vi "ListThisLevelDependencies.vi"(8 "error in (no error)":errorcluster, 11 "SMO in":refnum<class "SMO.lvclass">) -> (0 "error out":errorcluster, 2 "[My Dependencies]":refnum<class "SMO.lvclass">[](array[class]), 3 "SMO out":refnum<class "SMO.lvclass">)   [LabVIEW 2021, in "smo.lvlib" / "SMO.lvclass"]
uses:
  SMO.lvclass
  SMO.lvclass/SMO.ctl
  Private/GetDependencies.vi
  Support/Attribute.Dependencies/List Dependencies.vi
  Private/GetVariant(Attr).vi
  Private/ReftoDVR--SMO.vi
  Support/Attribute.Dependencies/Get GUIDs.vi
  isStateMachineObject.vi
  Support/Attribute.Dependencies/Attribute.Dependencies.lvclass
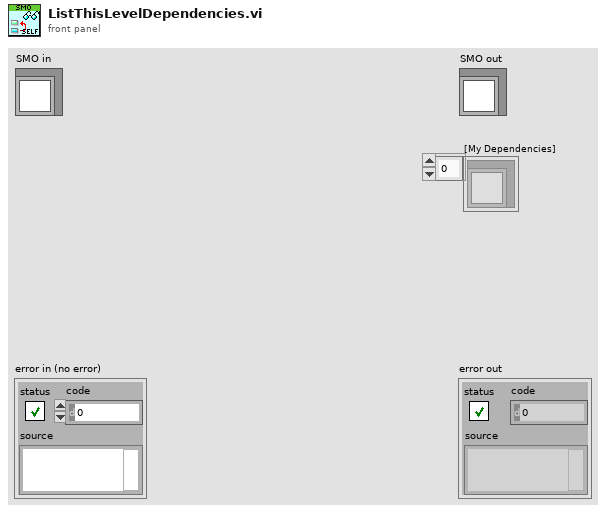
[diagram p1: front panel]
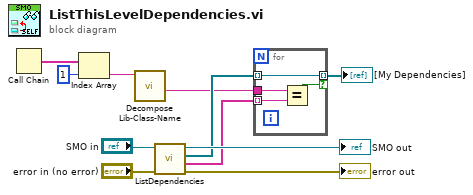
[diagram p0: block diagram]
diagram:
  n1 = Call Chain() -> (call chain=w11:string[])
  n2 = Index Array(array=w11, index=1) -> (element=w2:string)
  n3 = call "Decompose Lib-Class-Name.vi"("Qualified Name"=w2) -> ("className"=w1:string)  [unwired: 6 in, 4 out]
  n4 = call "ListDependencies.vi"("error in (no error)"="error in (no error)", "SMO in"="SMO in") -> ("error out"=→"error out":errorcluster, "Level"=w4:string[], "[Dependencies]"=w5:refnum<class "SMO.lvclass">[], "SMO out"=→"SMO out":refnum<class "SMO.lvclass">)  [unwired: 6 in]
  n5 = for {
    tunnel: [w15] -> w6 mode=indexing if=w14
    tunnel: w5 -> [w15] mode=indexing
    tunnel: w4 -> [w13] mode=indexing
    tunnel: w1 -> [w12]
    n6 = Equal?(x=w12, y=w13) -> (x = y?=w14:bool)
  }
  "[My Dependencies]" <- w6
